vi "Static Read.vi"(8 "error in (no error)":errorcluster, 11 "Abs_String in":refnum<class "Abs_String 1D.lvclass">) -> (0 "error out":errorcluster, 2 "Array":string[](array[string]), 3 "Abs_String out":refnum<class "Abs_String 1D.lvclass">)   [LabVIEW 2021, in "Abs_String 1D.lvclass"]
uses:
  Abs_String 1D.lvclass
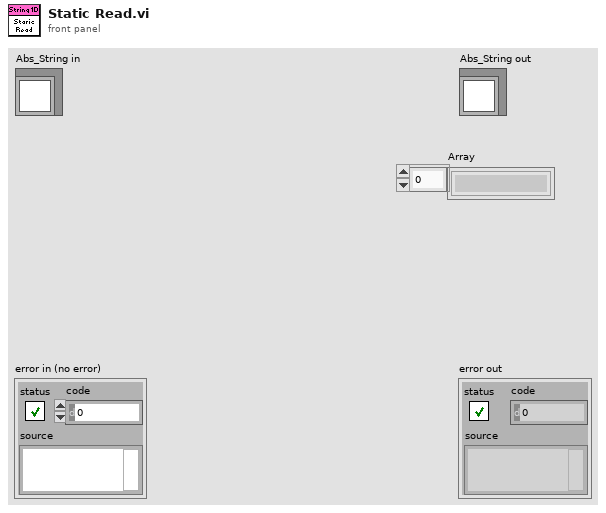
[diagram p1: front panel]
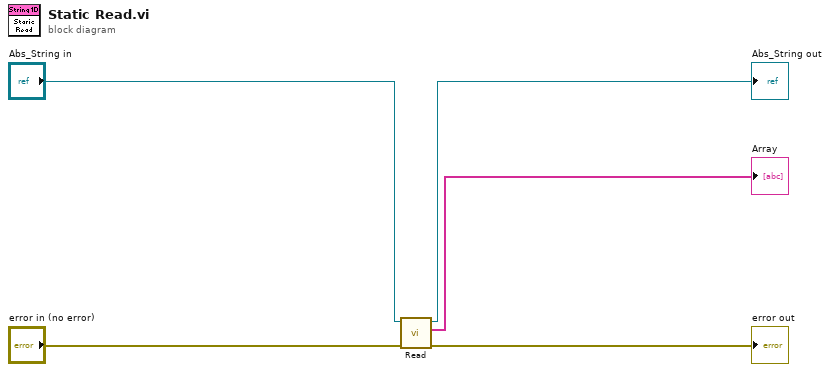
[diagram p0: block diagram]
diagram:
  n1 = call-dynamic "Read.vi"("error in (no error)"="error in (no error)", "Abs_String in"="Abs_String in") -> ("error out"=→"error out":errorcluster, "Array"=→"Array":string[], "Abs_String out"=→"Abs_String out":refnum<class "Abs_String 1D.lvclass">)  [unwired: 7 in]
